vi "Handle Error.vi"(8 "error in (no error)":errorcluster, 11 "Sim User Console Actor in":refnum<class "Sim User Console Actor.lvclass">) -> (0 "error out":errorcluster, 2 "stop actor?":bool=TRUE, 3 "Sim User Console Actor out":refnum<class "Sim User Console Actor.lvclass">)   [LabVIEW 2019, in "Sim User Console Actor.lvlib" / "Sim User Console Actor.lvclass"]
doc: "(<B>Filename</B>: Actor Framework.lvlib:Actor.lvclass:Handle Error.vi)\n\nDefines how the actor handles an error that occurred while processing a message. By default, this method does nothing except stop the actor."
uses:
  Sim User Console Actor.lvclass
  C:/Program Files (x86)/National Instruments/LabVIEW 2019/vi.lib/ActorFramework/Actor/Actor.lvclass
  ATM Controller/ATM Controller/Error Level.ctl
  <vilib>/ActorFramework/Actor/Actor.lvclass/Actor.ctl
  ATM Controller/ATM Controller Messages/Handle Error Msg/Handle Error Msg.lvclass/Handle Error Msg.ctl
  <vilib>/ActorFramework/Message Enqueuer/Message Enqueuer.lvclass/Message Enqueuer.ctl
  <vilib>/ActorFramework/Message Enqueuer/Enqueue.vi
  ATM Controller/ATM Controller Messages/Handle Error Msg/Handle Error Msg.lvclass
  C:/Program Files (x86)/National Instruments/LabVIEW 2019/vi.lib/ActorFramework/Message/Message.lvclass
  <vilib>/ActorFramework/Message Priority Queue/Priority Enqueue.vi
  User Console Actor/User Console Actor/User Console Actor.lvclass
  <vilib>/ActorFramework/Actor/Actor.lvclass
  ATM Controller/ATM Controller/ATM Controller.lvclass
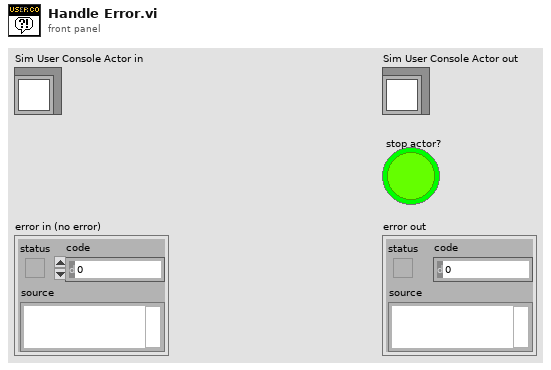
[diagram p1: front panel]
types:
  T1 = typedef "ATM Controller.lvlib/ATM Controller.lvclass/Error Level.ctl" = enum16{"Console Error", "Sensor Interface IO Error", "Process Step Error"}
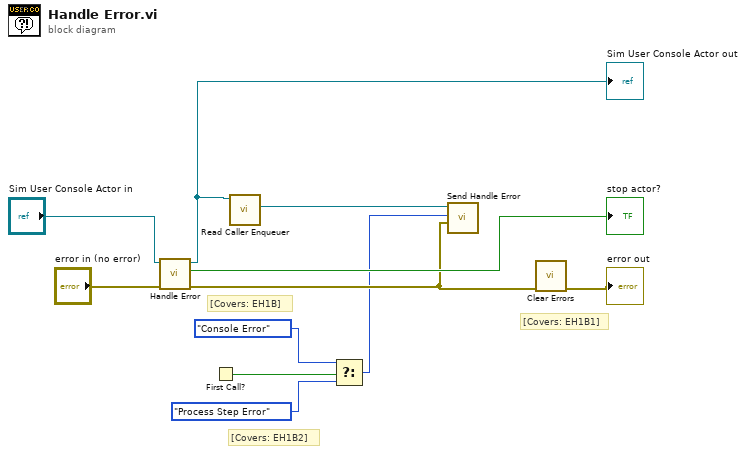
[diagram p0: block diagram]
diagram:
  # "[Covers: EH1B2]"
  # "[Covers: EH1B1]"
  # "[Covers: EH1B]"
  n1 = call-parent "Handle Error.vi"("error in (no error)"="error in (no error)", "Actor in"="Sim User Console Actor in") -> ("error out"=w6:errorcluster, "stop actor?"=→"stop actor?":bool, "Actor out"=w8:refnum<class "Sim User Console Actor.lvclass">)  [unwired: 7 in]
  "Sim User Console Actor out" <- w8
  n2 = First Call?() -> (First Call?: T/F=w3:bool)
  n3 = call <vilib>:"Read Caller Enqueuer.vi"("Actor"=w8) -> ("Caller Enqueuer"=w7:refnum<class "Message Enqueuer.lvclass">)  [unwired: 10 in]
  n4 = Select(t=Error_Level."Console Error" ("Error Level"), s=w3, f=Error_Level."Process Step Error" ("Error Level")) -> (s? t:f=w1:T1)
  n5 = call "Send Handle Error.vi"("Error"=w6, "Error Level"=w1, "Message Enqueuer"=w7) -> ()  [unwired: 7 in, 2 out]
  n6 = call <vilib>:"Clear Errors.vi"("error in (no error)"=w6) -> ("error out"=→"error out":errorcluster)  [unwired: 5 in, 1 out]
